vi "__get_level.vi"(2 "error in":errorcluster) -> (0 "error out":errorcluster, 1 "Current (mA)":dbl)   [LabVIEW 2013]
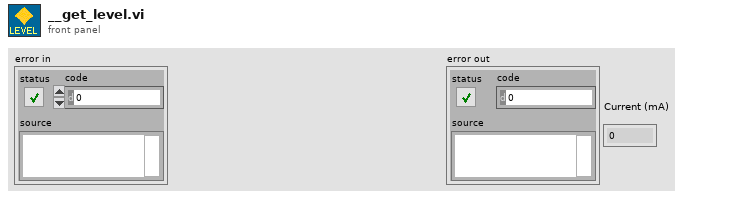
[diagram p1: front panel]
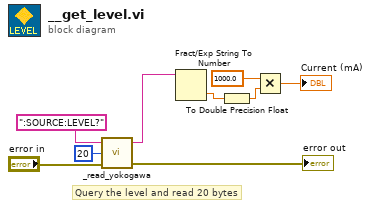
[diagram p0: block diagram]
diagram:
  # "Query the level and read 20 bytes"
  n1 = call "_read_yokogawa.vi"("error in"="error in", "Bytes to read"=u32 20, "Command to read"=":SOURCE:LEVEL?") -> ("error out"=→"error out":errorcluster, "Output"=w5:string)  [unwired: 1 in]
  n2 = Fract/Exp String To Number(string=w5) -> (number=w4:dbl)  [unwired: 3 in, 1 out]
  n3 = To Double Precision Float(number=w4) -> (double precision float=w3:dbl)
  n4 = Multiply(x=1000.0, y=w3) -> (x*y=→"Current (mA)":dbl)
